vi "PH_Numbers.Clockstring.vi"(0 "Time [s]":dbl) -> (1 "Clock String":string, 2 "<0?":bool)   [LabVIEW 2014, in "PH_Common.lvlib"]
doc: "This VI creates out of a double input a string. Input must be in seconds, so the output is of format HH:MM:ss."
uses:
  PH_Common.lvlib
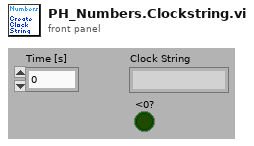
[diagram p1: front panel]
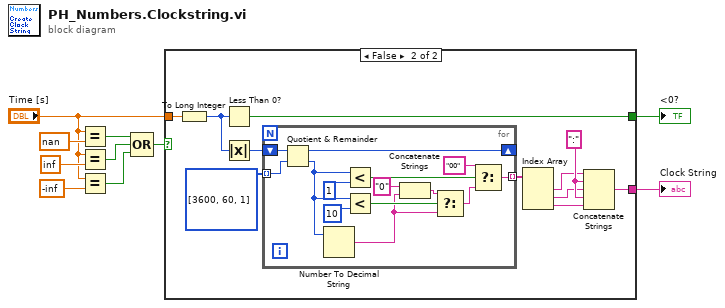
[diagram p0: block diagram]
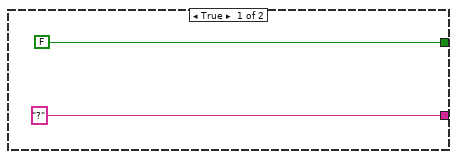
[diagram p2: hidden frame]
diagram:
  n1 = Equal?(x="Time [s]", y=nan) -> (x = y?=w6:bool)
  n2 = Equal?(x="Time [s]", y=inf) -> (x = y?=w5:bool)
  n3 = Equal?(x="Time [s]", y=-inf) -> (x = y?=w4:bool)
  n4 = Compound Arithmetic op=OR(w6, w5, w4) -> (w3:bool)
  n5 = case shown="False" w3 {
    tunnel: ["?" w13] -> w10
    tunnel: "Time [s]" -> [_ w23]
    tunnel: [FALSE w21] -> w1
    frame True {
    }
    frame False {
      w19 = ":" ("string")
      n6 = To Long Integer(number=w23) -> (32bit integer=w22:i32)
      n7 = Less Than 0?(x=w22) -> (x < 0?=w21:bool)
      n8 = Absolute Value(x=w22) -> (abs(x)=w20:i32)
      n9 = for {
        tunnel: i32[] [3600, 60, 1] -> [w26] mode=indexing
        tunnel: [w28] -> w17 mode=indexing
        shift-right: [w25] -> _
        shift-left: w20 -> [w27]
        n10 = Quotient & Remainder(x=w27, y=w26) -> (x-y*floor(x/y)=w25:i32, floor(x/y)=w24:i32)
        n11 = Number To Decimal String(number=w24) -> (decimal integer string=w29:string)  [unwired: 1 in]
        n12 = Less?(x=w24, y=1) -> (x < y?=w36:bool)
        n13 = Less?(x=w24, y=10) -> (x < y?=w33:bool)
        n14 = Concatenate Strings("0" ("string"), w29) -> (w30:string)
        n15 = Select(t=w30, s=w33, f=w29) -> (s? t:f=w32:string)
        n16 = Select(t="00" ("string"), s=w36, f=w32) -> (s? t:f=w28:string)
      }
      n17 = Index Array(array=w17) -> (element #1=w16:string, element #2=w15:string, element #3=w14:string)  [unwired: 3 in]
      n18 = Concatenate Strings(w16, w19, w15, w19, w14) -> (w13:string)
    }
  }
  "Clock String" <- w10
  "<0?" <- w1
